vi "Shooter M3.vi"(7 "Time Elapsed":bool, 8 "Hi":bool, 9 "Lo":bool, 10 "Disarm":bool, 11 "Fire Button":bool) -> (0 "3":enum16{"Unlock", "Lock"}(ring), 1 "2":enum16{"Enabled", "Retracted"}(ring), 2 "1":enum16{"Enabled", "Retracted"}(ring))   [LabVIEW 2013]
panel:
  out "Current State":string
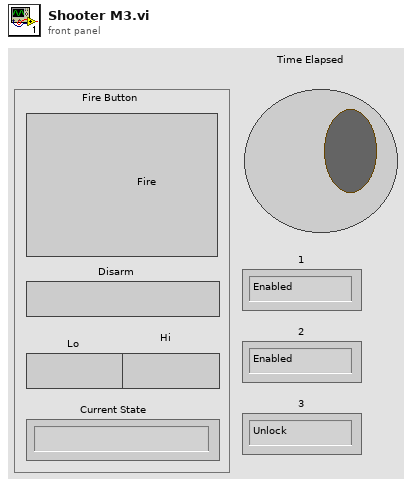
[diagram p1: front panel]
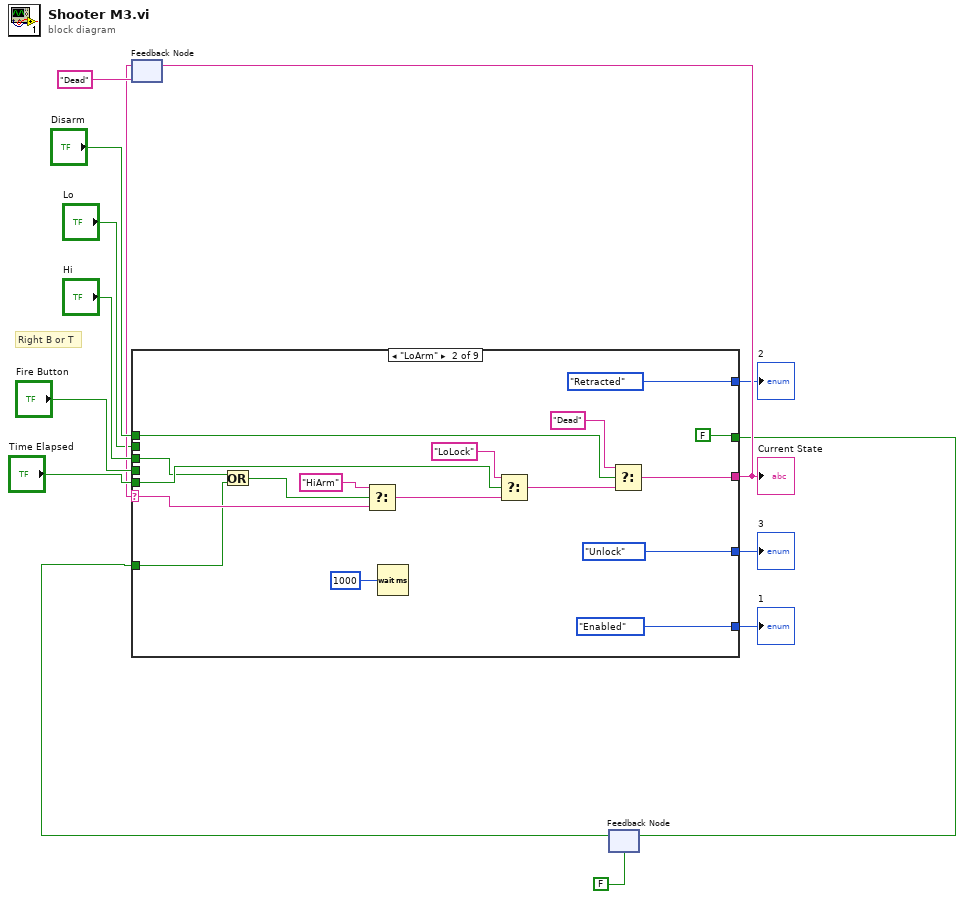
[diagram p0: block diagram]
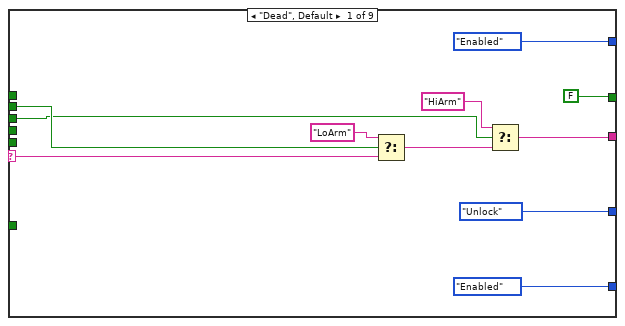
[diagram p2: hidden frame]
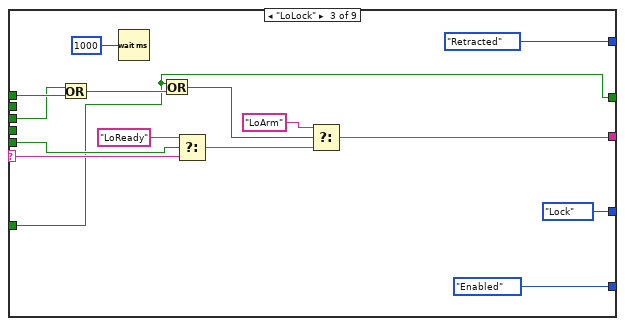
[diagram p3: hidden frame]
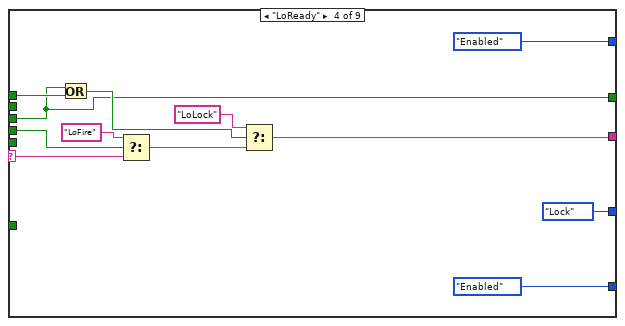
[diagram p4: hidden frame]
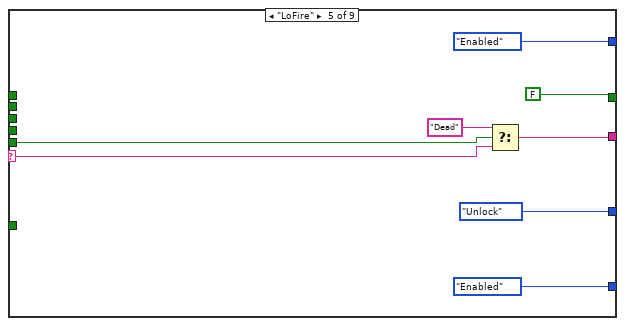
[diagram p5: hidden frame]
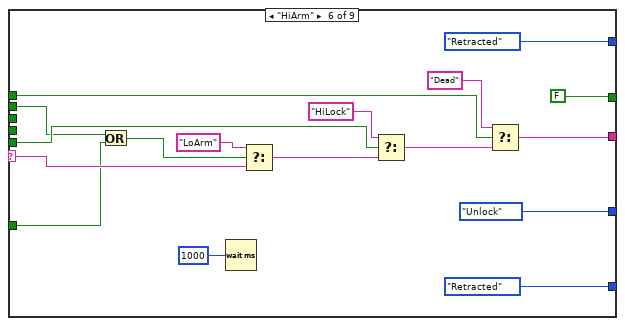
[diagram p6: hidden frame]
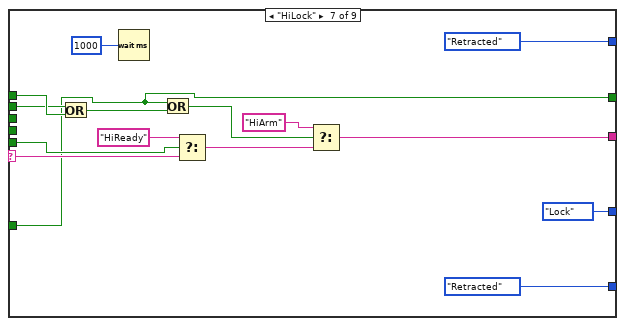
[diagram p7: hidden frame]
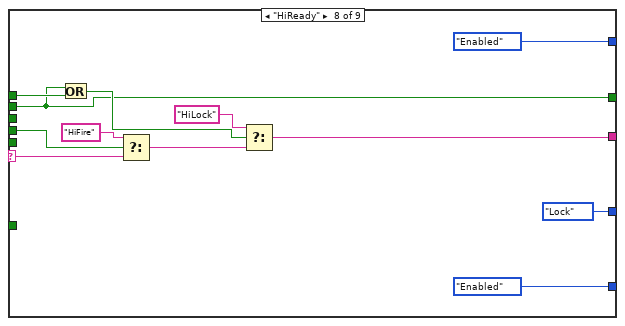
[diagram p8: hidden frame]
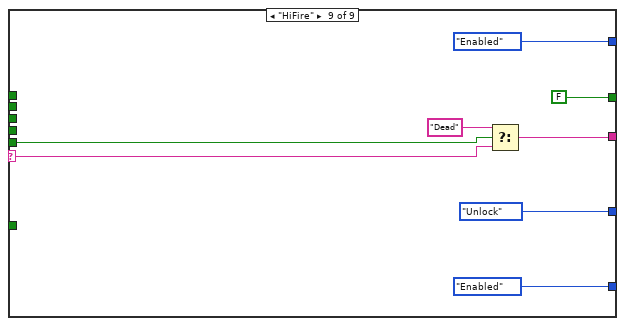
[diagram p9: hidden frame]
diagram:
  # "Right B or T"
  n1 = feedback #1("Dead") -> (w9:string)
  n2 = feedback #2(FALSE) -> (w2:bool)
  n3 = case shown="\"LoArm\"" w9 {
    selector: w9 -> [w22 w36 w52 w64 w77 w88 w107 w116 w126]
    tunnel: "Lo" -> [w24 _ _ _ _ w82 w103 w110 _]
    tunnel: "Hi" -> [w23 w29 w50 w58 _ _ _ _ _]
    tunnel: [w19 w40 w54 w65 w74 w86 w105 w117 w128] -> w8
    tunnel: "Disarm" -> [_ w42 w51 w62 _ w87 w104 w115 _]
    tunnel: "Time Elapsed" -> [_ w38 w53 _ w75 w89 w106 _ w127]
    tunnel: "Fire Button" -> [_ _ _ w66 _ _ _ w118 _]
    tunnel: [enum16{"Enabled", "Retracted"}."Enabled" enum16{"Enabled", "Retracted"}."Enabled" enum16{"Enabled", "Retracted"}."Enabled" enum16{"Enabled", "Retracted"}."Enabled" enum16{"Enabled", "Retracted"}."Enabled" enum16{"Enabled", "Retracted"}."Retracted" enum16{"Enabled", "Retracted"}."Retracted" enum16{"Enabled", "Retracted"}."Enabled" enum16{"Enabled", "Retracted"}."Enabled"] -> w7
    tunnel: [enum16{"Enabled", "Retracted"}."Enabled" enum16{"Enabled", "Retracted"}."Retracted" enum16{"Enabled", "Retracted"}."Retracted" enum16{"Enabled", "Retracted"}."Enabled" enum16{"Enabled", "Retracted"}."Enabled" enum16{"Enabled", "Retracted"}."Retracted" enum16{"Enabled", "Retracted"}."Retracted" enum16{"Enabled", "Retracted"}."Enabled" enum16{"Enabled", "Retracted"}."Enabled"] -> w6
    tunnel: [enum16{"Unlock", "Lock"}."Unlock" enum16{"Unlock", "Lock"}."Unlock" enum16{"Unlock", "Lock"}."Lock" enum16{"Unlock", "Lock"}."Lock" enum16{"Unlock", "Lock"}."Unlock" enum16{"Unlock", "Lock"}."Unlock" enum16{"Unlock", "Lock"}."Lock" enum16{"Unlock", "Lock"}."Lock" enum16{"Unlock", "Lock"}."Unlock"] -> w5
    tunnel: w2 -> [_ w28 w43 _ _ w80 w95 _ _]
    tunnel: [FALSE FALSE w43 w58 FALSE FALSE w95 w110 FALSE] -> w3
    frame "Dead", Default {
      n4 = Select(t="LoArm", s=w24, f=w22) -> (s? t:f=w25:string)
      n5 = Select(t="HiArm", s=w23, f=w25) -> (s? t:f=w19:string)
    }
    frame "LoArm" {
      n6 = Or(x=w29, y=w28) -> (x .or. y?=w30:bool)
      n7 = Select(t="HiArm", s=w30, f=w36) -> (s? t:f=w35:string)
      n8 = Wait (ms)(milliseconds to wait=u32 1000) -> ()  [unwired: 1 out]
      n9 = Select(t="LoLock", s=w38, f=w35) -> (s? t:f=w39:string)
      n10 = Select(t="Dead", s=w42, f=w39) -> (s? t:f=w40:string)
    }
    frame "LoLock" {
      n11 = Or(x=w50, y=w51) -> (x .or. y?=w44:bool)
      n12 = Wait (ms)(milliseconds to wait=u32 1000) -> ()  [unwired: 1 out]
      n13 = Or(x=w43, y=w44) -> (x .or. y?=w45:bool)
      n14 = Select(t="LoReady", s=w53, f=w52) -> (s? t:f=w56:string)
      n15 = Select(t="LoArm", s=w45, f=w56) -> (s? t:f=w54:string)
    }
    frame "LoReady" {
      n16 = Or(x=w58, y=w62) -> (x .or. y?=w63:bool)
      n17 = Select(t="LoFire", s=w66, f=w64) -> (s? t:f=w68:string)
      n18 = Select(t="LoLock", s=w63, f=w68) -> (s? t:f=w65:string)
    }
    frame "LoFire" {
      n19 = Select(t="Dead", s=w75, f=w77) -> (s? t:f=w74:string)
    }
    frame "HiArm" {
      n20 = Or(x=w82, y=w80) -> (x .or. y?=w81:bool)
      n21 = Wait (ms)(milliseconds to wait=u32 1000) -> ()  [unwired: 1 out]
      n22 = Select(t="LoArm", s=w81, f=w88) -> (s? t:f=w91:string)
      n23 = Select(t="HiLock", s=w89, f=w91) -> (s? t:f=w93:string)
      n24 = Select(t="Dead", s=w87, f=w93) -> (s? t:f=w86:string)
    }
    frame "HiLock" {
      n25 = Or(x=w103, y=w104) -> (x .or. y?=w96:bool)
      n26 = Wait (ms)(milliseconds to wait=u32 1000) -> ()  [unwired: 1 out]
      n27 = Or(x=w95, y=w96) -> (x .or. y?=w97:bool)
      n28 = Select(t="HiReady", s=w106, f=w107) -> (s? t:f=w108:string)
      n29 = Select(t="HiArm", s=w97, f=w108) -> (s? t:f=w105:string)
    }
    frame "HiReady" {
      n30 = Or(x=w110, y=w115) -> (x .or. y?=w114:bool)
      n31 = Select(t="HiFire", s=w118, f=w116) -> (s? t:f=w120:string)
      n32 = Select(t="HiLock", s=w114, f=w120) -> (s? t:f=w117:string)
    }
    frame "HiFire" {
      n33 = Select(t="Dead", s=w127, f=w126) -> (s? t:f=w128:string)
    }
  }
  "Current State" <- w8
  "1" <- w7
  "2" <- w6
  "3" <- w5
  n34 = feedback-in #1(w8) -> ()
  n35 = feedback-in #2(w3) -> ()
